vi "gun_speed_control P2IDv2.vi"(9 "Period (sec)":dbl, 10 "Speed (rps)":dbl, 11 "Gun Const":T1={"gun"={"num_lines"=0.0, "gain_kp1"=0.0, "gain_kp2"=0.0, "gain_ki"=0.0, "gain_kd"=0.0}, "turret"={"center_ana"=0.0, "volts_per_180"=0.0, "man_scale"=0.0, "turret_idg"={"low_fault_ana"=0.0, "high_fault_ana"=0.0, "min_ana"=0.0, "max_ana"=0.0, "movement_thresh"=0.0, "movement_time"=0.0}, "turret_pid"={"kP"=0.0, "kI"=0.0, "kD"=0.0}, "turret_invert"=TRUE, "turret_low_power"=0.0}, "tracking"={"velocity_lead_gain"=0.0, "velocity_rotation_gain"=0.0}, "hood"={"hood_idg"={"low_fault_ana"=0.0, "high_fault_ana"=0.0, "min_ana"=0.0, "max_ana"=0.0, "movement_thresh"=0.0, "movement_time"=0.0}, "hood_pid"={"kP"=0.0, "kI"=0.0, "kD"=0.0}, "hood_scale"={"min_ana"=0.0, "min_units"=0.0, "max_ana"=0.0, "max_units"=0.0}, "hood_invert"=FALSE}}) -> (1 "rpm raw":dbl, 2 "Sensor Speed (rps)":dbl, 3 "Output":dbl)   [LabVIEW 2011]
uses:
  gun_const_t.ctl
  gun_idg_const.ctl
  common/gain_const.ctl
  common/scale_const.ctl
  signals/Signal.ctl
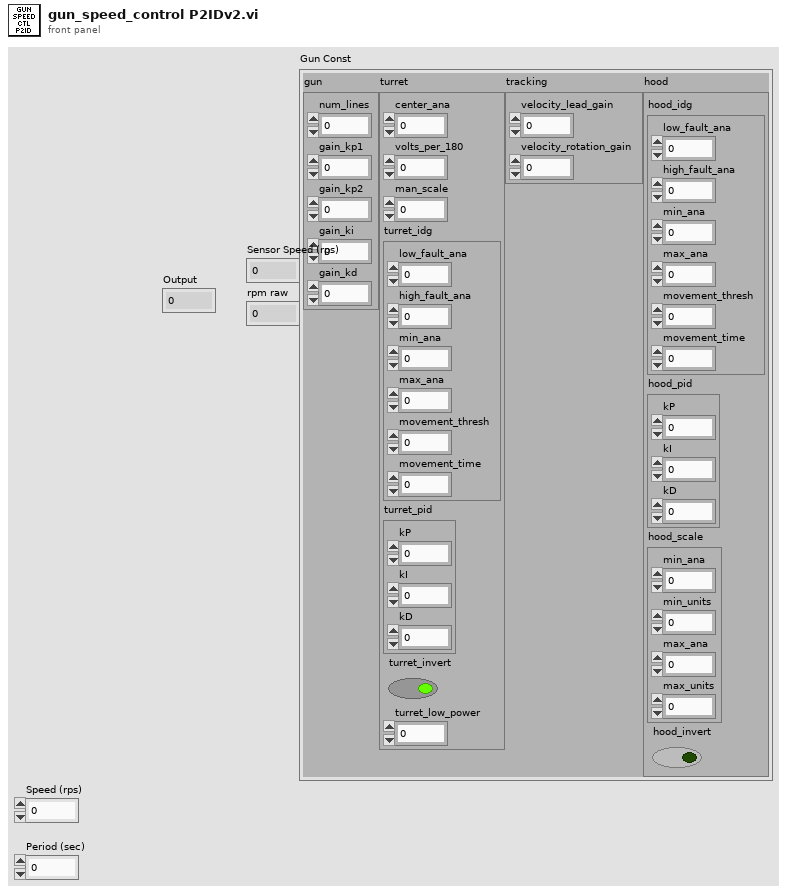
[diagram p1: front panel]
types:
  T1 = typedef "gun_const_t.ctl" = cluster{"gun":cluster{"num_lines":dbl, "gain_kp1":dbl, "gain_kp2":dbl, "gain_ki":dbl, "gain_kd":dbl}, "turret":cluster{"center_ana":dbl, "volts_per_180":dbl, "man_scale":dbl, "turret_idg":T2, "turret_pid":T3, "turret_invert":bool, "turret_low_power":dbl}, "tracking":cluster{"velocity_lead_gain":dbl, "velocity_rotation_gain":dbl}, "hood":cluster{"hood_idg":T2, "hood_pid":T3, "hood_scale":T4, "hood_invert":bool}}
  T2 = typedef "gun_idg_const.ctl" = cluster{"low_fault_ana":dbl, "high_fault_ana":dbl, "min_ana":dbl, "max_ana":dbl, "movement_thresh":dbl, "movement_time":dbl}
  T3 = typedef "gain_const.ctl" = cluster{"kP":dbl, "kI":dbl, "kD":dbl}
  T4 = typedef "scale_const.ctl" = cluster{"min_ana":dbl, "min_units":dbl, "max_ana":dbl, "max_units":dbl}
  T5 = typedef "Signal.ctl" = enum16{"SIGFIRE", "SIGSTOPSCRIPT", "SIGSTARTGUN", "SIGSTOPGUN", "SIGDISABLED", "SIGENABLED", "SIGUDPTIMEOUT", "SIGNEWVISION_REMOTE", "SIGNEWVISION_LOCAL", "SIGSHOTFIRED", "SIGDOTRACK", "SIGDONTTRACK"}
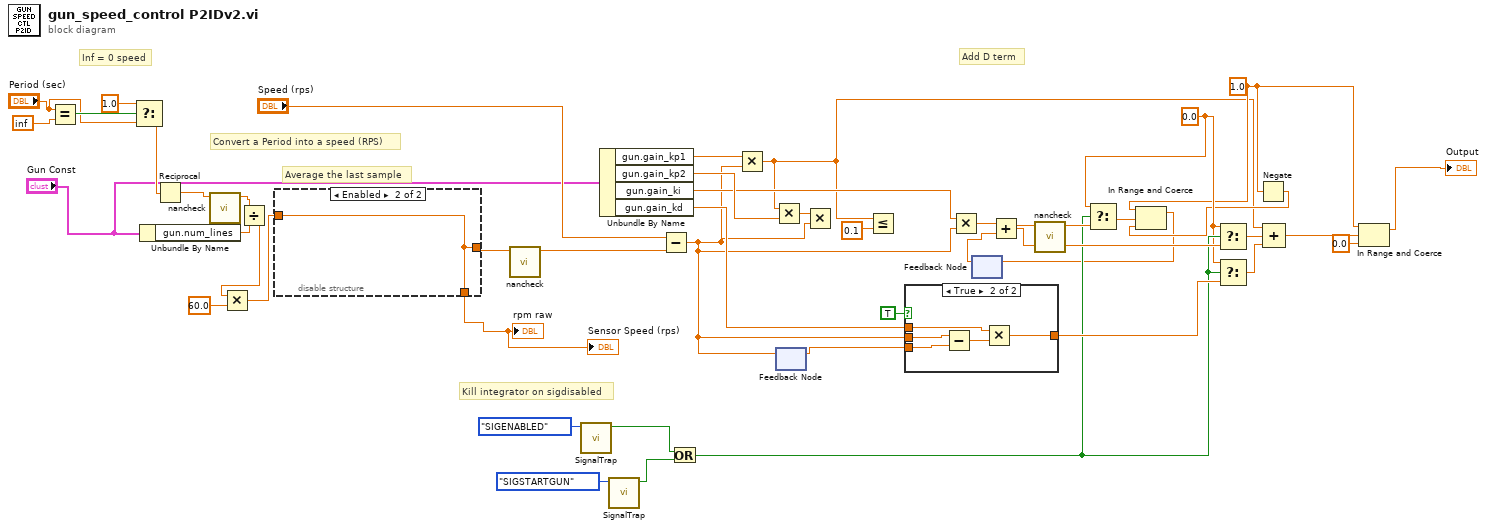
[diagram p0: block diagram]
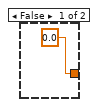
[diagram p2: hidden frame]
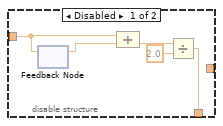
[diagram p3: hidden frame]
diagram:
  w8 = 0.0
  w6 = 1.0
  # "Add D term"
  # "Inf = 0 speed"
  # "Kill integrator on sigdisabled"
  # "Average the last sample"
  # "Convert a Period into a speed (RPS)"
  n1 = Equal?(x="Period (sec)", y=inf) -> (x = y?=w43:bool)
  n2 = Select(t=1.0, s=w43, f="Period (sec)") -> (s? t:f=w38:dbl)
  n3 = Unbundle By Name("Gun Const") -> ("gun.num_lines"=w46:dbl)
  n4 = Reciprocal(x=w38) -> (1/x=w39:dbl)
  n5 = call "nancheck.vi"("nancheck_in"=w39) -> ("nancheck_out"=w40:dbl)  [unwired: 10 in]
  n6 = Divide(x=w40, y=w46) -> (x/y=w33:dbl)
  n7 = Multiply(x=w33, y=60.0) -> (x*y=w34:dbl)
  n8 = disable-structure shown="Enabled" {
    disable-tunnel: w34 -> [w48 w52]
    disable-tunnel: [w47 w52] -> w11
    disable-tunnel: [_ w52] -> w15
    frame Disabled {
      n9 = feedback #1() -> (w49:dbl)  [unwired: 1 in]
      n10 = feedback-in #1(w48) -> ()
      n11 = Compound Arithmetic op=ADD(w48, w49) -> (w50:dbl)
      n12 = Divide(x=w50, y=2.0) -> (x/y=w47:dbl)
    }
    frame Enabled {
    }
  }
  "Sensor Speed (rps)" <- w11
  "rpm raw" <- w11
  n13 = call "nancheck.vi"("nancheck_in"=w15) -> ("nancheck_out"=w14:dbl)  [unwired: 10 in]
  n14 = call "SignalTrap.vi"("Signal"=Signal."SIGENABLED") -> ("Trapped Signal"=w36:bool)  [unwired: 10 in]
  n15 = Unbundle By Name("Gun Const") -> ("gun.gain_kp1"=w31:dbl, "gun.gain_kp2"=w24:dbl, "gun.gain_ki"=w20:dbl, "gun.gain_kd"=w28:dbl)
  n16 = call "SignalTrap.vi"("Signal"=Signal."SIGSTARTGUN") -> ("Trapped Signal"=w35:bool)  [unwired: 10 in]
  n17 = Subtract(x="Speed (rps)", y=w14) -> (x-y=w19:dbl)
  n18 = Or(x=w36, y=w35) -> (x .or. y?=w9:bool)
  n19 = Multiply(x=w31, y=w19) -> (x*y=w2:dbl)
  n20 = Multiply(x=w2, y=w24) -> (x*y=w12:dbl)
  n21 = feedback #2() -> (w23:dbl)  [unwired: 1 in]
  n22 = feedback-in #2(w19) -> ()
  n23 = Multiply(x=w12, y=w19) -> ()  [unwired: 1 out]
  n24 = Less Or Equal?(x=w2, y=0.1) -> ()  [unwired: 1 out]
  n25 = case shown="True" TRUE {
    tunnel: [0.0 w56] -> w25
    tunnel: w19 -> [_ w54]
    tunnel: w28 -> [_ w57]
    tunnel: w23 -> [_ w55]
    frame False {
    }
    frame True {
      n26 = Subtract(x=w54, y=w55) -> (x-y=w58:dbl)
      n27 = Multiply(x=w57, y=w58) -> (x*y=w56:dbl)
    }
  }
  n28 = Multiply(x=w20, y=w19) -> (x*y=w22:dbl)
  n29 = feedback #3() -> (w21:dbl)  [unwired: 1 in]
  n30 = Add(x=w22, y=w21) -> (x+y=w13:dbl)
  n31 = call "nancheck.vi"("nancheck_in"=w13) -> ("nancheck_out"=w10:dbl)  [unwired: 10 in]
  n32 = Select(t=w8, s=w9, f=w10) -> (s? t:f=w7:dbl)
  n33 = Select(t=w8, s=w9, f=w13) -> (s? t:f=w27:dbl)
  n34 = Select(t=w8, s=w9, f=w25) -> (s? t:f=w26:dbl)
  n35 = Negate(x=w6) -> (-x=w5:dbl)
  n36 = In Range and Coerce(upper limit=w6, x=w7, lower limit=w5) -> (coerced(x)=w4:dbl)  [unwired: 1 out]
  n37 = feedback-in #3(w4) -> ()
  n38 = Compound Arithmetic op=ADD(w2, w27, w26) -> (w29:dbl)
  n39 = In Range and Coerce(upper limit=w6, x=w29, lower limit=0.0) -> (coerced(x)=→"Output":dbl)  [unwired: 1 out]
